vi "MAT Read Matrix.vi"(0 "Ref Num":refnum<file>, 2 "variable offset in (-1: current position)":i64=-1, 3 "first matrix column (0: first one)":i32, 4 "maximum matrix columns (-1: all)":i32=-1, 5 "Error In":errorcluster) -> (6 "Matrix Name":string, 8 "Representation":T1, 9 "CSG":csg[][](array[numeric]) format="%.2f", 10 "STR":string[](array[string]), 11 "CDB":cdb[][](array[numeric]) format="%.2f", 12 "DBL":dbl[][](array[numeric]) format="%.2f", 13 "U8":u8[][](array[numeric]), 14 "Dup Ref Num":refnum<file>, 15 "SGL":sgl[][](array[numeric]) format="%.2f", 16 "I32":i32[][](array[numeric]), 17 "I16":i16[][](array[numeric]), 18 "U16":u16[][](array[numeric]), 19 "error out":errorcluster)   [LabVIEW 2018]
doc: "\"Save to MAT\" saves a 2D array of numbers or a 1D array of strings to MATLAB file. It works only with LabVIEW for Windows. All data types, described in MATLAB/External Interface Guide/Appendix A, are supported, except Sparse Matrices.\n\nAll data inputs should be 2D arrays, except String input which should be a 1D array. Only one data input may contain a non-empty array, otherwise error will be generated (error code -1).\n\nSAVML.LLB is a freeware written by Serge Liberman <liber@us1.channel1.com>."
uses:
  MAT Type Representation.ctl
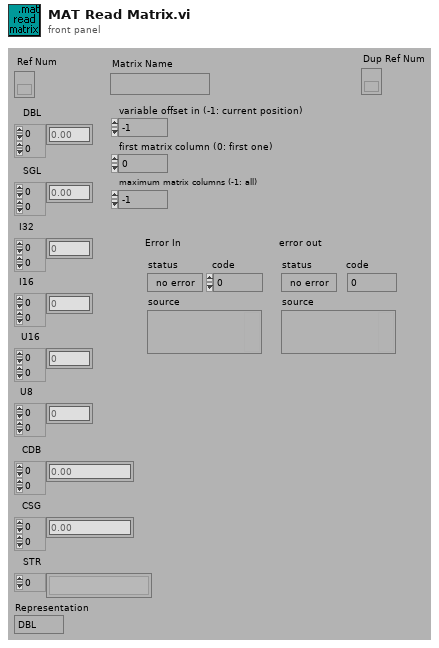
[diagram p1: front panel]
types:
  T1 = typedef "MAT Type Representation.ctl" = enum16{"DBL", "SGL", "I32", "I16", "U16", "U8", "CDB", "CSG", "STR"}
  T2 = enum16{"big-endian, network order", "native, host order", "little-endian"}
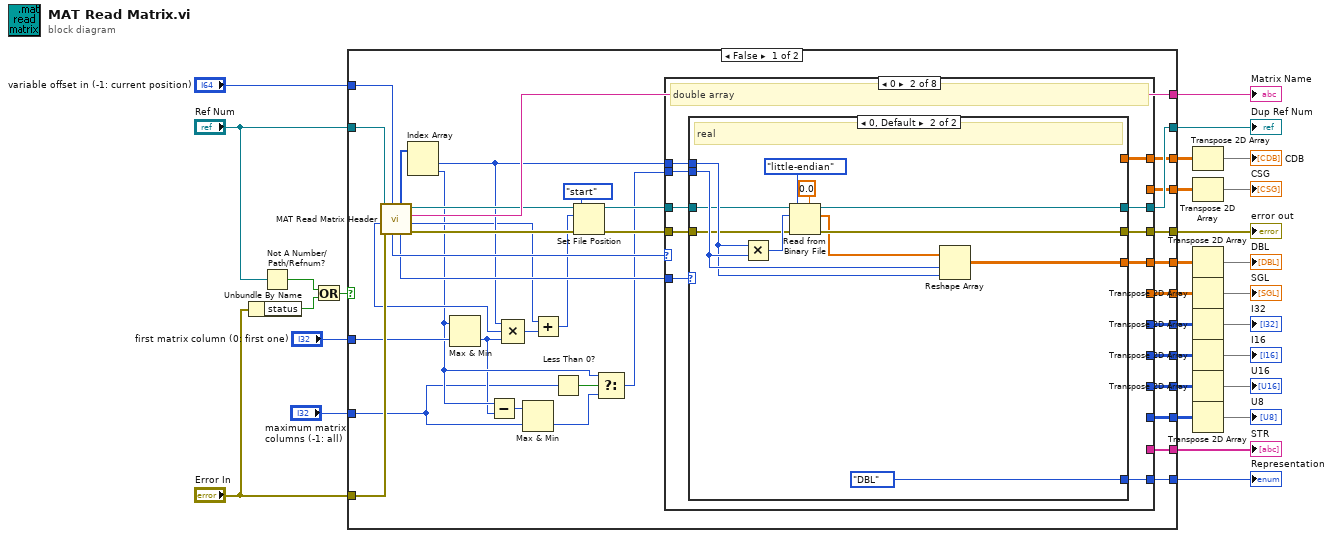
[diagram p0: block diagram]
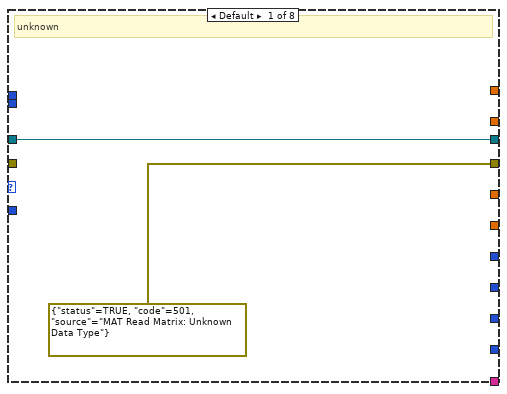
[diagram p2: hidden frame]
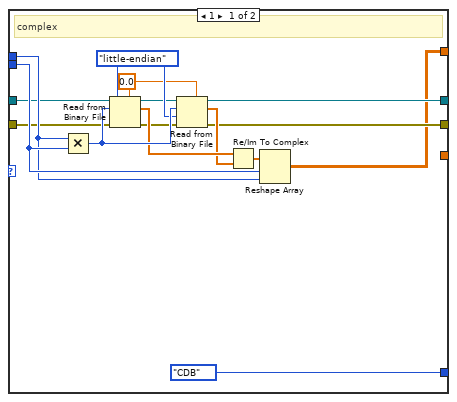
[diagram p3: hidden frame]
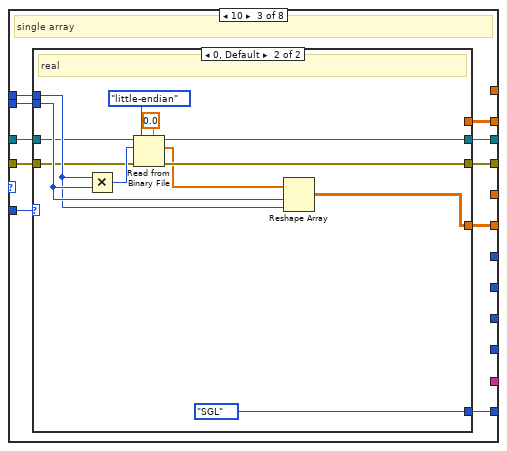
[diagram p4: hidden frame]
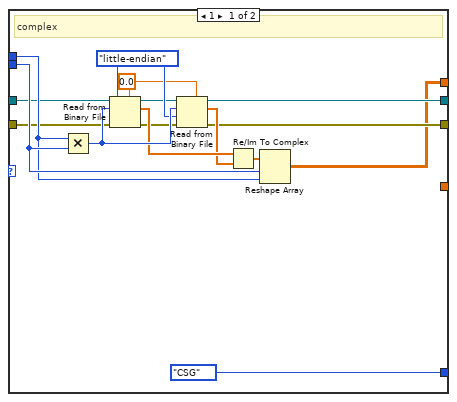
[diagram p5: hidden frame]
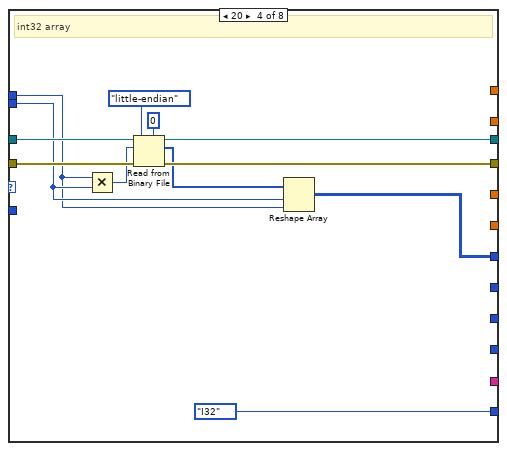
[diagram p6: hidden frame]
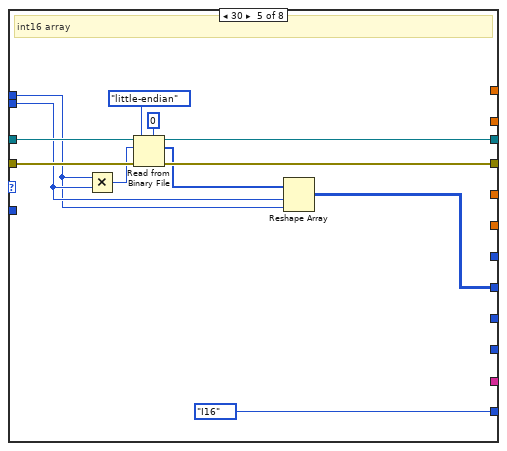
[diagram p7: hidden frame]
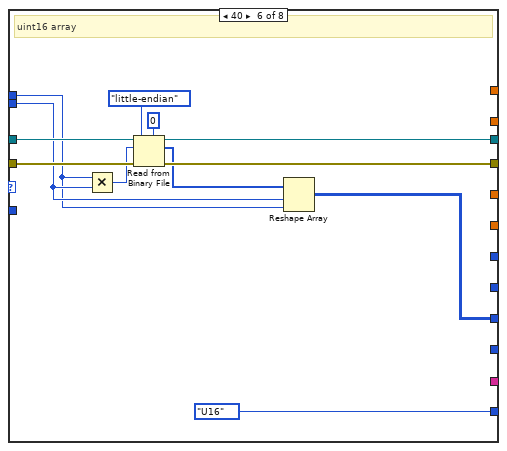
[diagram p8: hidden frame]
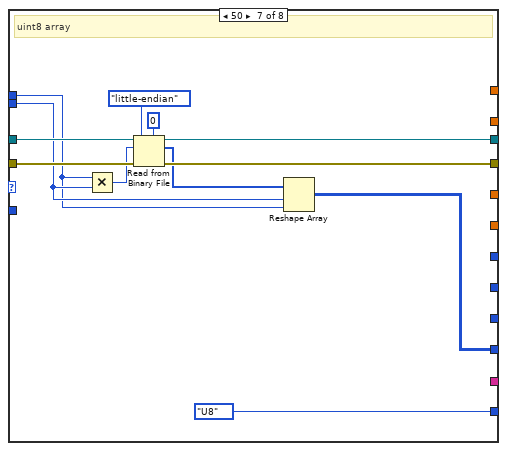
[diagram p9: hidden frame]
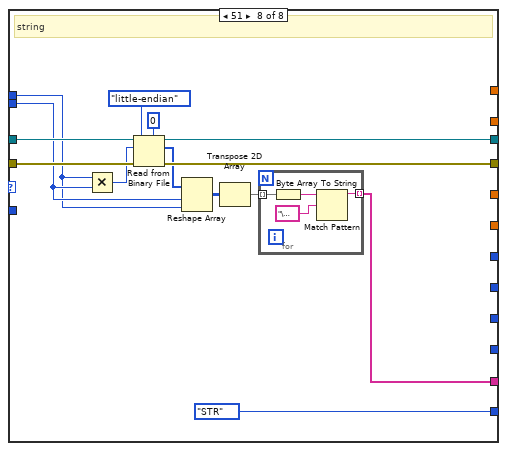
[diagram p10: hidden frame]
diagram:
  n1 = Unbundle By Name("Error In") -> ("status"=w26:bool)
  n2 = Not A Number/Path/Refnum?(number/path/refnum="Ref Num") -> (NaN/Path/Refnum?=w24:bool)
  n3 = Or(x=w24, y=w26) -> (x .or. y?=w23:bool)
  n4 = case shown="False" w23 {
    tunnel: [w66 w212] -> w29
    tunnel: "Ref Num" -> [w64 w212]
    tunnel: "Error In" -> [w50 w211]
    tunnel: [w65 w211] -> w27
    tunnel: [w62 _] -> w22
    tunnel: [w61 _] -> w21
    tunnel: [w60 _] -> w20
    tunnel: [w59 _] -> w19
    tunnel: [w57 _] -> w18
    tunnel: [w56 _] -> w17
    tunnel: [w55 _] -> w16
    tunnel: [w54 _] -> w15
    tunnel: [w53 _] -> w14
    tunnel: [w52 _] -> w6
    tunnel: [w51 _] -> w13
    tunnel: "variable offset in (-1: current position)" -> [w43 _]
    tunnel: "first matrix column (0: first one)" -> [w42 _]
    tunnel: "maximum matrix columns (-1: all)" -> [w31 _]
    frame False {
      n5 = call "MAT Read Matrix Header.vi"("offset in (-1: current position)"=w43, "Error In"=w50, "Ref Num"=w64) -> ("error out"=w47:errorcluster, "data offset out"=w38:i64, "Matrix Name"=w62:string, "Dup Ref Num"=w46:refnum<file>, "Real/Complex (0 - Real)"=w58:u32, "Matrix Size (rows x cols)"=w44:i32[], "Rep. Code"=w63:u32, "element byte size"=w41:i32)  [unwired: 1 out]
      n6 = Index Array(array=w44) -> (element #1=w40:i32, element #2=w34:i32)  [unwired: 2 in]
      n7 = Max & Min(x=w34, y=w42) -> (min(x,y)=w32:i32)  [unwired: 1 out]
      n8 = Subtract(x=w34, y=w32) -> (x-y=w36:i32)
      n9 = Compound Arithmetic op=MULTIPLY(w40, w41, w32) -> (w39:i32)
      n10 = Max & Min(x=w36, y=w31) -> (min(x,y)=w30:i32)  [unwired: 1 out]
      n11 = Add(x=w38, y=w39) -> (x+y=w37:i64)
      n12 = Less Than 0?(x=w31) -> (x < 0?=w35:bool)
      n13 = Set File Position(offset (in bytes) (0)=w37, refnum=w46, from (0:start)=enum16{"start", "end", "current"}."start", error in=w47) -> (refnum out=w48:refnum<file>, error out=w49:errorcluster)
      n14 = Select(t=w34, s=w35, f=w30) -> (s? t:f=w33:i32)
      n15 = case shown="0" w63 {
        tunnel: w48 -> [w68 w78 w116 w156 w168 w180 w192 w206]
        tunnel: [w68 w77 w115 w155 w167 w179 w191 w205] -> w66
        tunnel: w49 -> [_ w75 w113 w153 w165 w177 w189 w203]
        tunnel: [errorcluster {"status"=TRUE, "code"=501, "source"="MAT Read Matrix: Unknown Data Type"} ("error in (no error)") w76 w114 w154 w166 w178 w190 w204] -> w65
        tunnel: [_ w74 w112 MAT_Type_Representation."I32" ("Representation") MAT_Type_Representation."I16" ("Representation") MAT_Type_Representation."U16" ("Representation") MAT_Type_Representation."U8" ("Representation") MAT_Type_Representation."STR" ("Representation")] -> w61
        tunnel: w33 -> [_ w73 w111 w151 w163 w175 w187 w201]
        tunnel: w40 -> [_ w72 w110 w150 w162 w174 w186 w200]
        tunnel: [_ w71 _ _ _ _ _ _] -> w60
        tunnel: [_ _ w107 _ _ _ _ _] -> w59
        tunnel: w58 -> [_ w70 w109 _ _ _ _ _]
        tunnel: [_ _ _ w145 _ _ _ _] -> w57
        tunnel: [_ _ _ _ w157 _ _ _] -> w56
        tunnel: [_ _ _ _ _ w169 _ _] -> w55
        tunnel: [_ _ _ _ _ _ w181 _] -> w54
        tunnel: [_ _ _ _ _ _ _ w193] -> w53
        tunnel: [_ w69 _ _ _ _ _ _] -> w52
        tunnel: [_ _ w108 _ _ _ _ _] -> w51
        frame Default {
          # "unknown"
        }
        frame 0 {
          # "double array"
          n16 = case shown="0, Default" w70 {
            tunnel: w78 -> [w80 w99]
            tunnel: [w86 w97] -> w77
            tunnel: [w87 w98] -> w76
            tunnel: w75 -> [w81 w100]
            tunnel: [MAT_Type_Representation."CDB" ("Representation") MAT_Type_Representation."DBL" ("Representation")] -> w74
            tunnel: w73 -> [w85 w102]
            tunnel: w72 -> [w84 w101]
            tunnel: [_ w95] -> w71
            tunnel: [w79 _] -> w69
            frame 1 {
              w92 = T2."little-endian" ("byte order (0:big-endian, network order)")
              w91 = 0.0
              # "complex"
              n17 = Multiply(x=w84, y=w85) -> (x*y=w93:i32)
              n18 = Read from Binary File(5:w91, 8:w81, 9:w92, 10:w93, 11:w80) -> (0:w83:errorcluster, 2:w90:dbl[], 3:w82:refnum<file>)  [unwired: 1 in, 1 out]
              n19 = Read from Binary File(5:w91, 8:w83, 9:w92, 10:w93, 11:w82) -> (0:w87:errorcluster, 2:w89:dbl[], 3:w86:refnum<file>)  [unwired: 1 in, 1 out]
              n20 = Re/Im To Complex(1:w89, 2:w90) -> (0:w88:cdb[])
              n21 = Reshape Array(w88, w85, w84) -> (w79:cdb[][])
            }
            frame 0, Default {
              # "real"
              n22 = Multiply(x=w101, y=w102) -> (x*y=w105:i32)
              n23 = Read from Binary File(5:0.0, 8:w100, 9:T2."little-endian" ("byte order (0:big-endian, network order)"), 10:w105, 11:w99) -> (0:w98:errorcluster, 2:w96:dbl[], 3:w97:refnum<file>)  [unwired: 1 in, 1 out]
              n24 = Reshape Array(w96, w102, w101) -> (w95:dbl[][])
            }
          }
        }
        frame 10 {
          # "single array"
          n25 = case shown="0, Default" w109 {
            tunnel: w116 -> [w118 w137]
            tunnel: [w124 w135] -> w115
            tunnel: [w125 w136] -> w114
            tunnel: w113 -> [w119 w138]
            tunnel: [MAT_Type_Representation."CSG" ("Representation") MAT_Type_Representation."SGL" ("Representation")] -> w112
            tunnel: w111 -> [w123 w140]
            tunnel: w110 -> [w122 w139]
            tunnel: [w117 _] -> w108
            tunnel: [_ w133] -> w107
            frame 1 {
              w130 = T2."little-endian" ("byte order (0:big-endian, network order)")
              w129 = sgl 0.0
              # "complex"
              n26 = Multiply(x=w122, y=w123) -> (x*y=w131:i32)
              n27 = Read from Binary File(5:w129, 8:w119, 9:w130, 10:w131, 11:w118) -> (0:w121:errorcluster, 2:w128:sgl[], 3:w120:refnum<file>)  [unwired: 1 in, 1 out]
              n28 = Read from Binary File(5:w129, 8:w121, 9:w130, 10:w131, 11:w120) -> (0:w125:errorcluster, 2:w127:sgl[], 3:w124:refnum<file>)  [unwired: 1 in, 1 out]
              n29 = Re/Im To Complex(1:w127, 2:w128) -> (0:w126:csg[])
              n30 = Reshape Array(w126, w123, w122) -> (w117:csg[][])
            }
            frame 0, Default {
              # "real"
              n31 = Multiply(x=w139, y=w140) -> (x*y=w143:i32)
              n32 = Read from Binary File(5:sgl 0.0, 8:w138, 9:T2."little-endian" ("byte order (0:big-endian, network order)"), 10:w143, 11:w137) -> (0:w136:errorcluster, 2:w134:sgl[], 3:w135:refnum<file>)  [unwired: 1 in, 1 out]
              n33 = Reshape Array(w134, w140, w139) -> (w133:sgl[][])
            }
          }
        }
        frame 20 {
          # "int32 array"
          n34 = Multiply(x=w150, y=w151) -> (x*y=w149:i32)
          n35 = Read from Binary File(5:0, 8:w153, 9:T2."little-endian" ("byte order (0:big-endian, network order)"), 10:w149, 11:w156) -> (0:w154:errorcluster, 2:w146:i32[], 3:w155:refnum<file>)  [unwired: 1 in, 1 out]
          n36 = Reshape Array(w146, w151, w150) -> (w145:i32[][])
        }
        frame 30 {
          # "int16 array"
          n37 = Multiply(x=w162, y=w163) -> (x*y=w161:i32)
          n38 = Read from Binary File(5:i16 0, 8:w165, 9:T2."little-endian" ("byte order (0:big-endian, network order)"), 10:w161, 11:w168) -> (0:w166:errorcluster, 2:w158:i16[], 3:w167:refnum<file>)  [unwired: 1 in, 1 out]
          n39 = Reshape Array(w158, w163, w162) -> (w157:i16[][])
        }
        frame 40 {
          # "uint16 array"
          n40 = Multiply(x=w174, y=w175) -> (x*y=w173:i32)
          n41 = Read from Binary File(5:u16 0, 8:w177, 9:T2."little-endian" ("byte order (0:big-endian, network order)"), 10:w173, 11:w180) -> (0:w178:errorcluster, 2:w170:u16[], 3:w179:refnum<file>)  [unwired: 1 in, 1 out]
          n42 = Reshape Array(w170, w175, w174) -> (w169:u16[][])
        }
        frame 50 {
          # "uint8 array"
          n43 = Multiply(x=w186, y=w187) -> (x*y=w185:i32)
          n44 = Read from Binary File(5:u8 0, 8:w189, 9:T2."little-endian" ("byte order (0:big-endian, network order)"), 10:w185, 11:w192) -> (0:w190:errorcluster, 2:w182:u8[], 3:w191:refnum<file>)  [unwired: 1 in, 1 out]
          n45 = Reshape Array(w182, w187, w186) -> (w181:u8[][])
        }
        frame 51 {
          # "string"
          n46 = Multiply(x=w200, y=w201) -> (x*y=w199:i32)
          n47 = Read from Binary File(5:u8 0, 8:w203, 9:T2."little-endian" ("byte order (0:big-endian, network order)"), 10:w199, 11:w206) -> (0:w204:errorcluster, 2:w196:u8[], 3:w205:refnum<file>)  [unwired: 1 in, 1 out]
          n48 = Reshape Array(w196, w201, w200) -> (w195:u8[][])
          n49 = Transpose 2D Array(2D array=w195) -> (transposed array=w194:u8[][])
          n50 = for {
            tunnel: w194 -> [w210] mode=indexing
            tunnel: [w207] -> w193 mode=indexing
            n51 = Byte Array To String(unsigned byte array=w210) -> (string=w208:string)
            n52 = Match Pattern(string=w208, regular expression="\u0000") -> (before substring=w207:string)  [unwired: 1 in, 3 out]
          }
        }
      }
    }
    frame True {
    }
  }
  "error out" <- w27
  "Dup Ref Num" <- w29
  "Matrix Name" <- w22
  "Representation" <- w21
  "STR" <- w14
  n53 = Transpose 2D Array(2D array=w6) -> (transposed array=→"CDB":cdb[][])
  n54 = Transpose 2D Array(2D array=w13) -> (transposed array=→"CSG":csg[][])
  n55 = Transpose 2D Array(2D array=w20) -> (transposed array=→"DBL":dbl[][])
  n56 = Transpose 2D Array(2D array=w19) -> (transposed array=→"SGL":sgl[][])
  n57 = Transpose 2D Array(2D array=w18) -> (transposed array=→"I32":i32[][])
  n58 = Transpose 2D Array(2D array=w17) -> (transposed array=→"I16":i16[][])
  n59 = Transpose 2D Array(2D array=w16) -> (transposed array=→"U16":u16[][])
  n60 = Transpose 2D Array(2D array=w15) -> (transposed array=→"U8":u8[][])
